vi "ImagesPool.vi"(4 "Image":enum16{"Ups", "Downs", "Diffs", "Expands"}(ring), 6 "Op":T2=enum."Get Image", 7 "N Levels (12)":i32=12, 8 "error in (no error)":errorcluster) -> (0 "error out":errorcluster, 2 "Filtered Copy":T1, 3 "Array of Images":T1[](array[typedef]))   [LabVIEW 2023]
uses:
  ImagesPool Operations TypeDef.ctl
  <vilib>/vision/Image Controls.llb/IMAQ Image.ctl
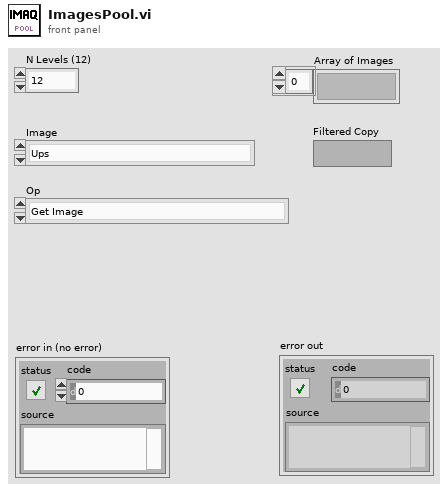
[diagram p1: front panel]
types:
  T1 = typedef "IMAQ Image.ctl" = refnum<image>
  T2 = typedef "ImagesPool Operations TypeDef.ctl" = enum16{"Init", "Get Image", "Dispose"}
  T3 = typedef "Image Type" = u32
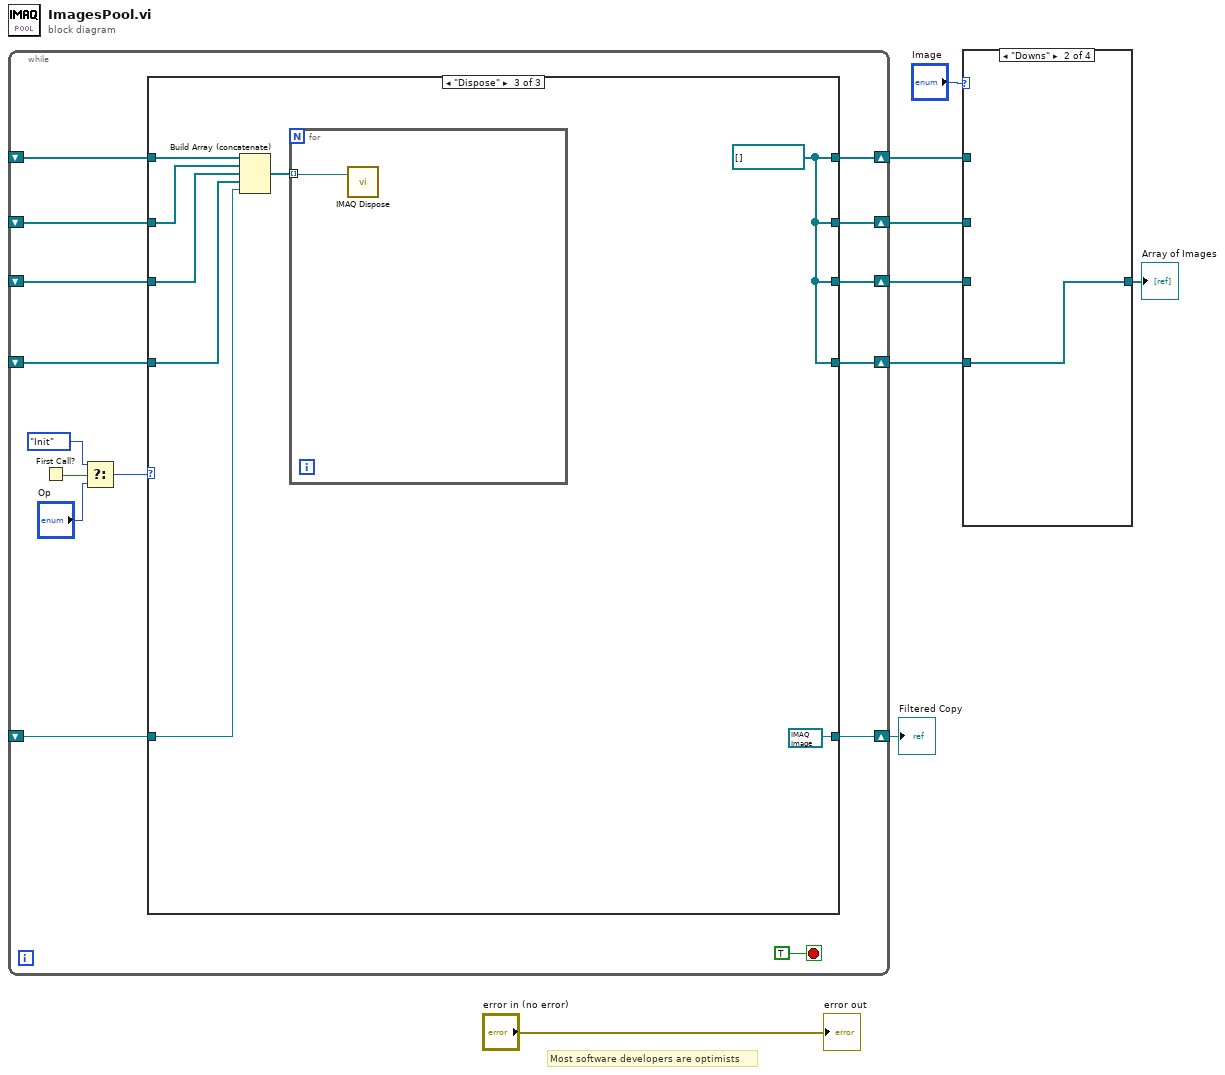
[diagram p0: block diagram]
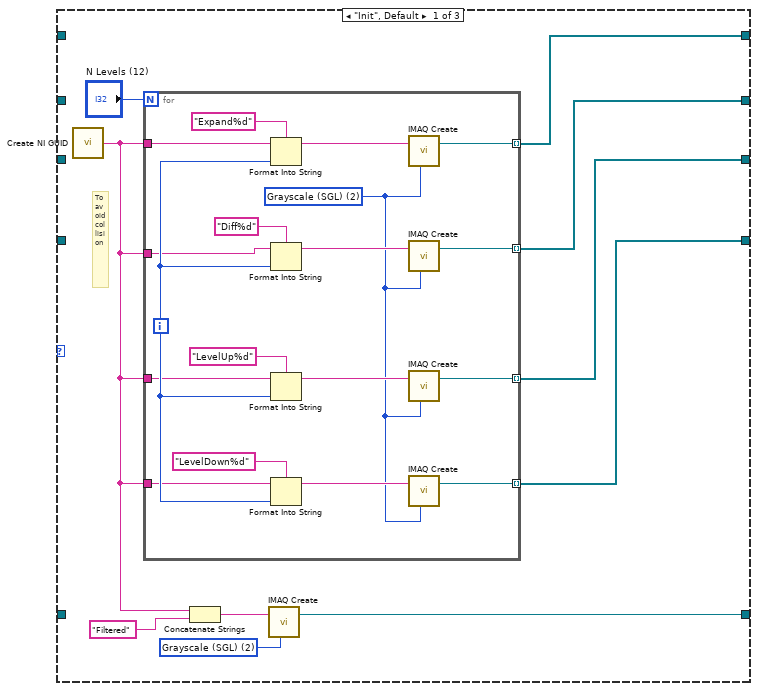
[diagram p5: hidden frame]
diagram:
  # "Most software developers are optimists"
  n1 = while {
    shift-right: [w22] -> w7
    shift-left: _ -> [w18]
    shift-right: [w21] -> w6
    shift-left: _ -> [w17]
    shift-right: [w20] -> w5
    shift-left: _ -> [w16]
    shift-right: [w19] -> w4
    shift-left: _ -> [w15]
    shift-right: [w10] -> w1
    shift-left: _ -> [w9]
    stop <- TRUE stop-if-true
    n2 = First Call?() -> (First Call?: T/F=w14:bool)
    n3 = Select(t=ImagesPool_Operations_TypeDef."Init", s=w14, f="Op") -> (s? t:f=w12:T2)
    n4 = case shown="\"Dispose\"" w12 {
      tunnel: [w32 w56 w63] -> w22
      tunnel: [w31 w55 w63] -> w21
      tunnel: [w30 w54 w63] -> w20
      tunnel: [w29 w53 w63] -> w19
      tunnel: w18 -> [_ w56 w62]
      tunnel: w17 -> [_ w55 w61]
      tunnel: w16 -> [_ w54 w60]
      tunnel: w15 -> [_ w53 w59]
      tunnel: [w26 w52 T1 refnum ("New Image")] -> w10
      tunnel: w9 -> [_ w52 w57]
      frame "Init", Default {
        w27 = T3 2 items=["Grayscale (U8)", "Grayscale (I16)", "Grayscale (SGL)", "Complex (CSG)", "RGB (U32)", "HSL (U32)", "RGB (U64)", "Grayscale (U16)"] ("Image Type")
        # "To avoid collision"
        n5 = call <vilib>:"Create NI GUID.vi"() -> ("NI GUID"=w24:string)
        n6 = for {
          N: "N Levels (12)" -> [_]
          tunnel: [w49] -> w29 mode=indexing
          tunnel: [w46] -> w30 mode=indexing
          tunnel: [w43] -> w31 mode=indexing
          tunnel: [w39] -> w32 mode=indexing
          tunnel: w24 -> [w37]
          tunnel: w24 -> [w36]
          tunnel: w24 -> [w35]
          tunnel: w24 -> [w34]
          i -> [w40]
          w38 = T3 2 items=["Grayscale (U8)", "Grayscale (I16)", "Grayscale (SGL)", "Complex (CSG)", "RGB (U32)", "HSL (U32)", "RGB (U64)", "Grayscale (U16)"] ("Image Type")
          n7 = Format Into String(format string="Expand%d", initial string=w37, w40) -> (resulting string=w42:string)  [unwired: 1 in, 1 out]
          n8 = Format Into String(format string="Diff%d", initial string=w36, w40) -> (resulting string=w44:string)  [unwired: 1 in, 1 out]
          n9 = Format Into String(format string="LevelUp%d", initial string=w35, w40) -> (resulting string=w48:string)  [unwired: 1 in, 1 out]
          n10 = Format Into String(format string="LevelDown%d", initial string=w34, w40) -> (resulting string=w51:string)  [unwired: 1 in, 1 out]
          n11 = call "IMAQ Create"("Image Name"=w42, "Image Type"=w38) -> ("New Image"=w39:T1)  [unwired: 3 in, 1 out]
          n12 = call "IMAQ Create"("Image Name"=w44, "Image Type"=w38) -> ("New Image"=w43:T1)  [unwired: 3 in, 1 out]
          n13 = call "IMAQ Create"("Image Name"=w48, "Image Type"=w38) -> ("New Image"=w46:T1)  [unwired: 3 in, 1 out]
          n14 = call "IMAQ Create"("Image Name"=w51, "Image Type"=w38) -> ("New Image"=w49:T1)  [unwired: 3 in, 1 out]
        }
        n15 = Concatenate Strings(w24, "Filtered" ("Image Name")) -> (w25:string)
        n16 = call "IMAQ Create"("Image Name"=w25, "Image Type"=w27) -> ("New Image"=w26:T1)  [unwired: 3 in, 1 out]
      }
      frame "Get Image" {
      }
      frame "Dispose" {
        w63 = T1[] []
        n17 = Build Array (concatenate)(w62, w61, w60, w59, w57) -> (w58:T1[])
        n18 = for {
          tunnel: w58 -> [w65] mode=indexing
          n19 = call "IMAQ Dispose"("Image"=w65) -> ()  [unwired: 5 in, 1 out]
        }
      }
    }
  }
  "Filtered Copy" <- w1
  n20 = case shown="\"Downs\"" "Image" {
    tunnel: w7 -> [_ _ _ w69]
    tunnel: w6 -> [_ _ w68 _]
    tunnel: w5 -> [w66 _ _ _]
    tunnel: w4 -> [_ w67 _ _]
    tunnel: [w66 w67 w68 w69] -> w3
    frame "Ups" {
    }
    frame "Downs" {
    }
    frame "Diffs" {
    }
    frame "Expands" {
    }
  }
  "Array of Images" <- w3
  "error out" <- "error in (no error)"
